vi "normal to hex string.vi"(11 "Normal String":string="Hello World!") -> (3 "Hex Display Sting":string)   [LabVIEW 2017]
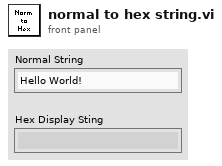
[diagram p1: front panel]
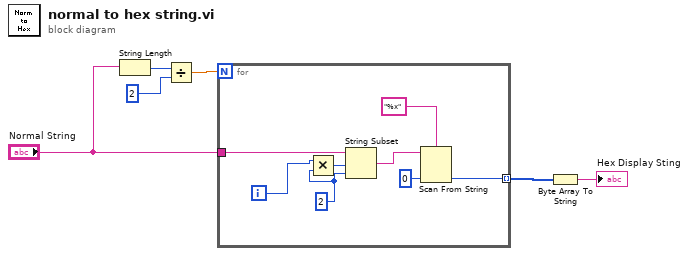
[diagram p0: block diagram]
diagram:
  n1 = String Length(string="Normal String") -> (length=w4:i32)
  n2 = Divide(x=w4, y=2) -> (x/y=w2:dbl)
  n3 = for {
    N: w2 -> [_]
    tunnel: "Normal String" -> [w12]
    tunnel: [w8] -> w1 mode=indexing
    i -> [w7]
    w9 = 2 ("length (rest)")
    n4 = Multiply(x=w7, y=w9) -> (x*y=w10:i32)
    n5 = String Subset(string=w12, offset (0)=w10, length (rest)=w9) -> (substring=w11:string)
    n6 = Scan From String(format string="%x", input string=w11, default 1=u8 0 ("default value 1")) -> (output 1=w8:u8)  [unwired: 2 in, 3 out]
  }
  n7 = Byte Array To String(unsigned byte array=w1) -> (string=→"Hex Display Sting":string)
